vi "Variant To Tree Map.vi"(11 "Children":variant) -> (1 "Tree Map (Empty)":T1, 2 "Empty?":bool, 3 "Children":variant)   [LabVIEW 2020, in "Blue Tree Map OpenSource.lvlib"]
uses:
  Blue Tree Map OpenSource.lvlib
  Typedefs/Tree Map.ctl
  Typedefs/Tree Map Data.ctl
  Typedefs/Tree Node Data.ctl
  Typedefs/Attribute Map.ctl
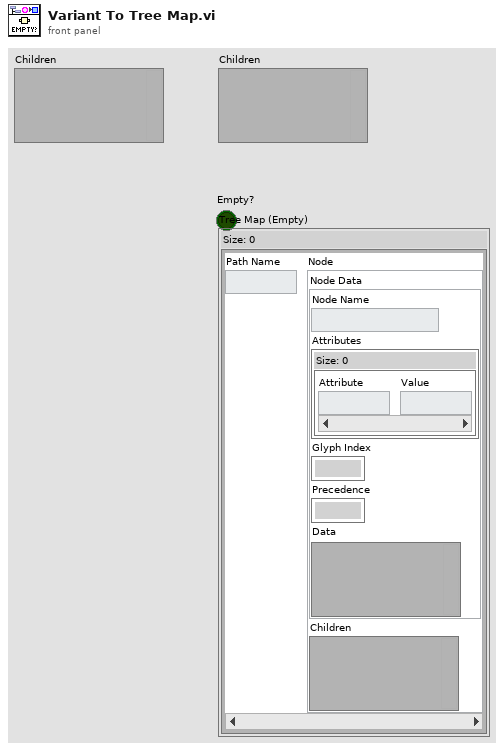
[diagram p1: front panel]
types:
  T1 = typedef "Blue Tree Map OpenSource.lvlib/Tree Map.ctl" = map{string, T2}
  T2 = typedef "Blue Tree Map OpenSource.lvlib/Tree Map Data.ctl" = cluster{"Node Data":T3, "Children":variant}
  T3 = typedef "Blue Tree Map OpenSource.lvlib/Tree Node Data.ctl" = cluster{"Node Name":string, "Attributes":T4, "Glyph Index":i32, "Precedence":i32, "Data":variant}
  T4 = typedef "Blue Tree Map OpenSource.lvlib/Attribute Map.ctl" = map{string, string}
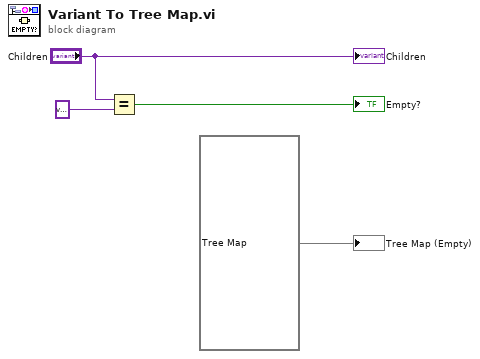
[diagram p0: block diagram]
diagram:
  n1 = Equal?(x="Children", y=variant ("Children")) -> (x = y?=→"Empty?":bool)
  "Tree Map (Empty)" <- T1 {} ("Tree Map Out")
  "Children" <- "Children"
